vi "str to int16.vi"(2 "String":string) -> (6 "int16":i16)   [LabVIEW 2014, in "OPCUA XML.lvlib"]
uses:
  OPCUA XML.lvlib
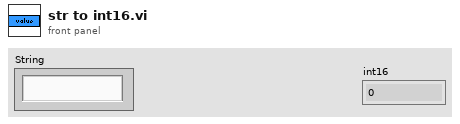
[diagram p1: front panel]
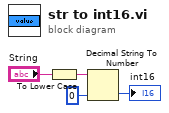
[diagram p0: block diagram]
diagram:
  n1 = To Lower Case(string="String") -> (all lower case string=w3:string)
  n2 = Decimal String To Number(string=w3, default (0L)=i16 0 ("default (0 I32)")) -> (number=→"int16":i16)  [unwired: 1 in, 1 out]
